vi "CheckSpeedSettings.vi"(2 "TB IP ADDRESS":string="192.168.0.100", 3 "CC IP ADDRESS":string="192.168.0.34", 4 "connection ID CC":refnum<k5>) -> (0 "PASS":bool, 1 "String 2":string)   [LabVIEW 2013]
panel:
  # "INPUTS"
  # "OUTPUTS"
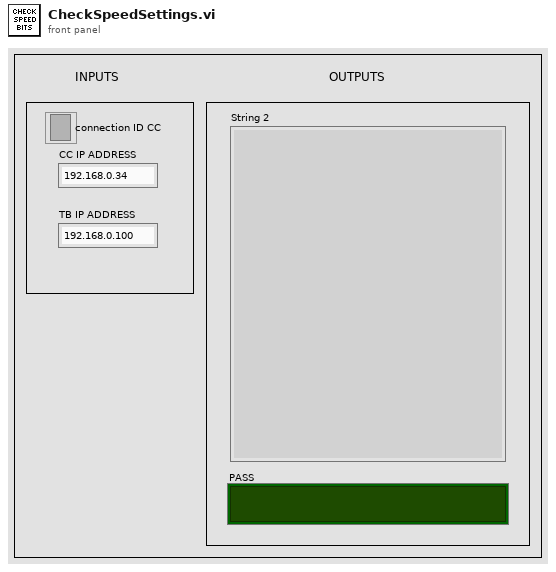
[diagram p1: front panel]
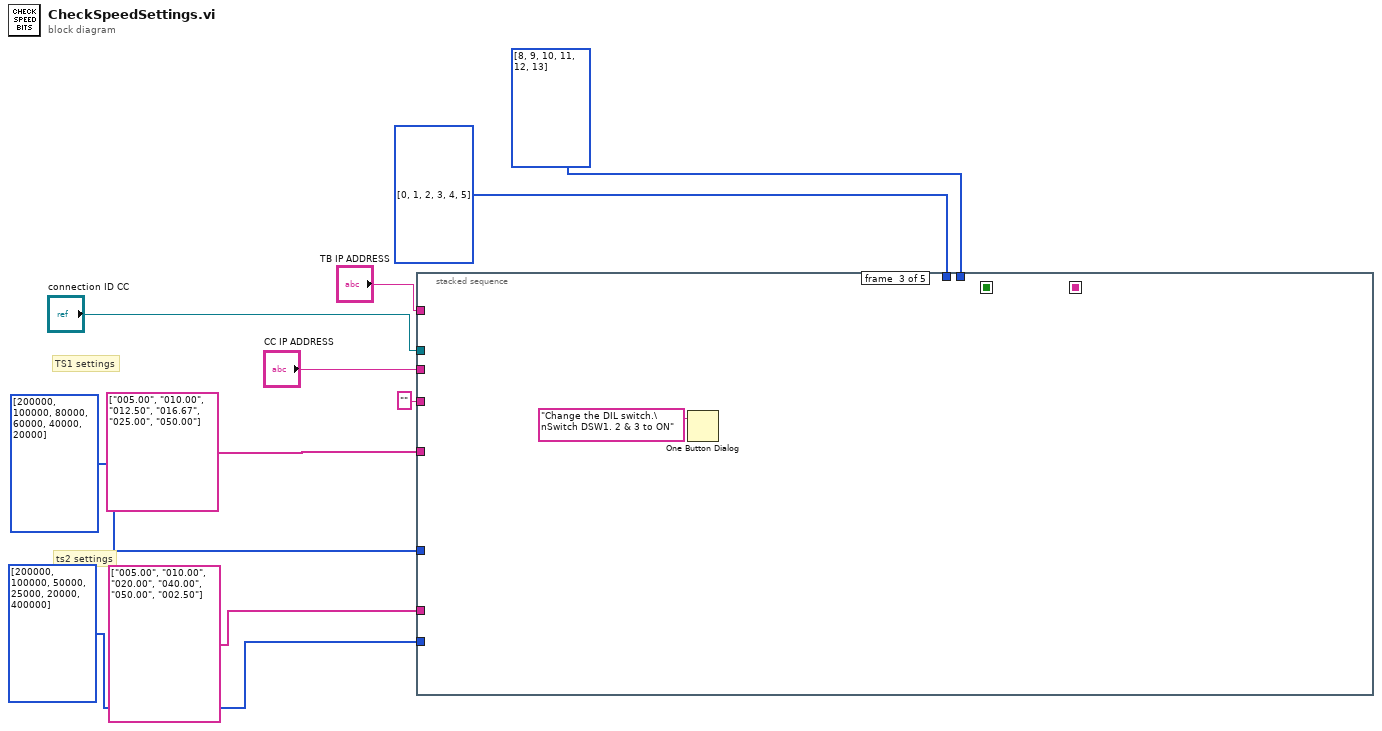
[diagram p0: block diagram]
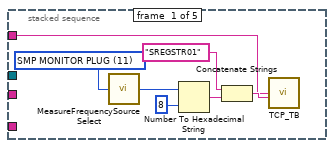
[diagram p2: hidden frame]
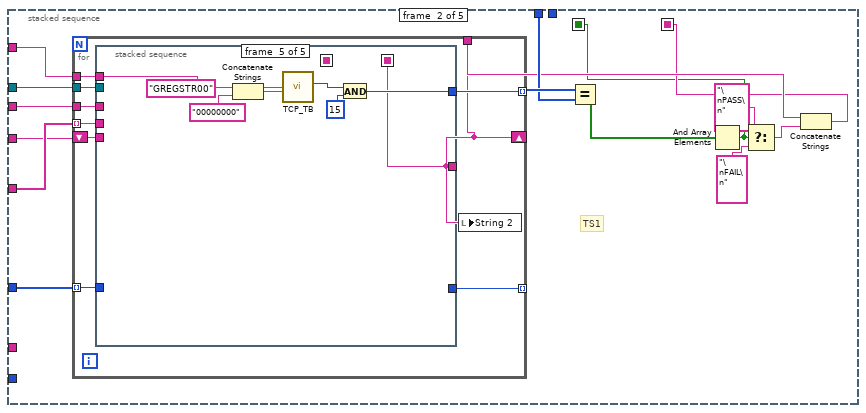
[diagram p3: hidden frame]
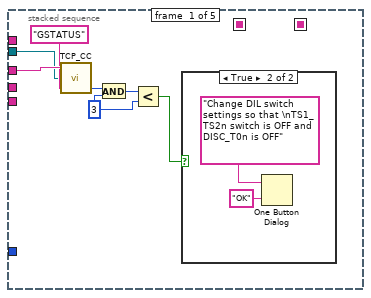
[diagram p4: hidden frame]
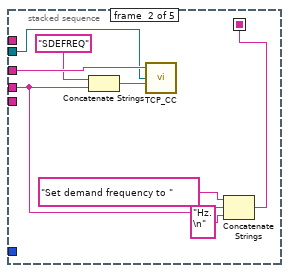
[diagram p6: hidden frame]
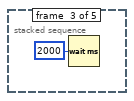
[diagram p7: hidden frame]
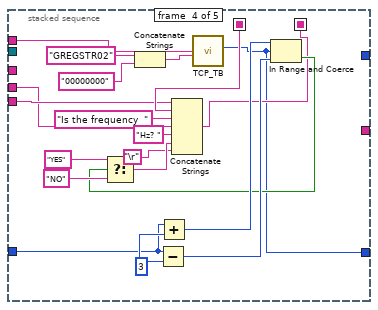
[diagram p8: hidden frame]
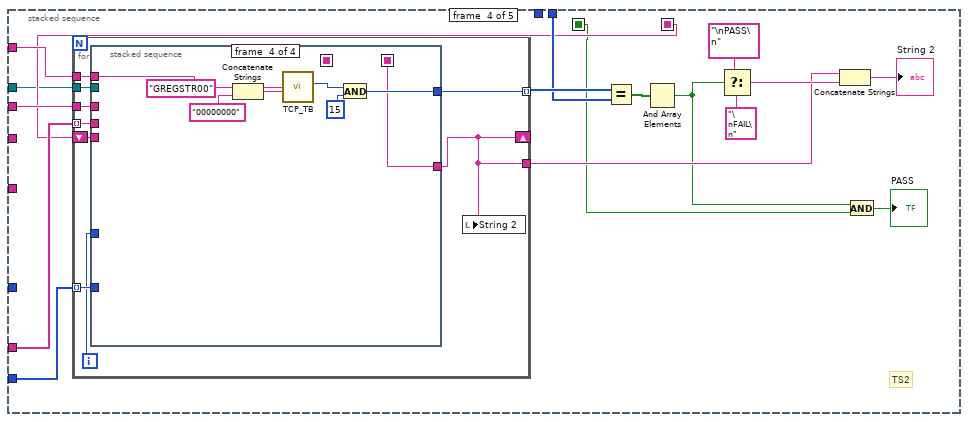
[diagram p9: hidden frame]
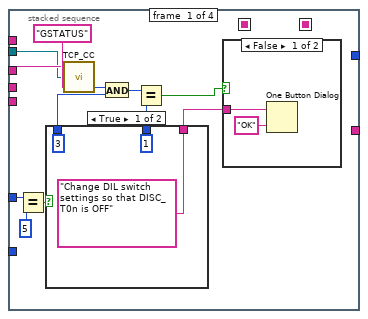
[diagram p10: hidden frame]
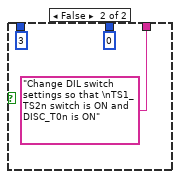
[diagram p11: hidden frame]
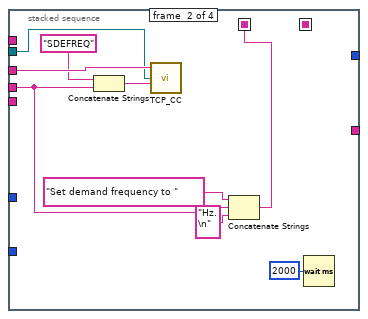
[diagram p13: hidden frame]
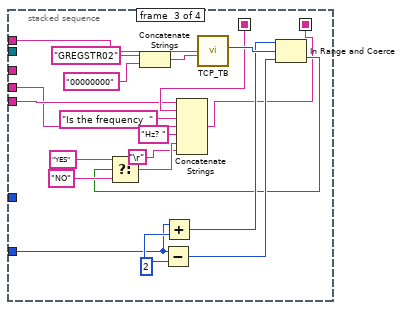
[diagram p14: hidden frame]
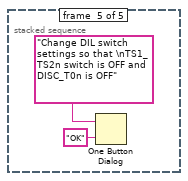
[diagram p15: hidden frame]
diagram:
  # "ts2 settings"
  # "TS1 settings"
  n1 = stacked-sequence {
    seq-local: [_ w20 _ _ _] -> [_ _ _ w99 _]
    seq-local: [_ w19 _ _ _] -> [_ _ _ w91 _]
    tunnel: "CC IP ADDRESS" -> [_ w32 _ w105 _]
    tunnel: "TB IP ADDRESS" -> [w11 w30 _ w104 _]
    tunnel: string[] ["005.00", "010.00", "012.50", "016.67", "025.00", "050.00"] -> [_ w31 _ _ _]
    tunnel: "" ("TB IP ADDRESS") -> [_ w29 _ _ _]
    tunnel: i32[] [200000, 100000, 80000, 60000, 40000, 20000] -> [_ w28 _ _ _]
    tunnel: u32[] [0, 1, 2, 3, 4, 5] ("Array") -> [_ w26 _ _ _]
    tunnel: string[] ["005.00", "010.00", "020.00", "040.00", "050.00", "002.50"] -> [_ _ _ w102 _]
    tunnel: i32[] [200000, 100000, 50000, 25000, 20000, 400000] -> [_ _ _ w101 _]
    tunnel: u32[] [8, 9, 10, 11, 12, 13] ("Array") -> [_ _ _ w100 _]
    tunnel: "connection ID CC" -> [_ w18 _ w89 _]
    frame #0 {
      w13 = u16 11 items=["1Mhz", "1MHz MONITOR PLUG", "DSMP", "DSMP MONITOR PLUG", "RP", "RP MONITOR PLUG", "MP", "MP MONITOR PLUG", "EEP 1.2 Sec", "EEP MONITOR PLUG", "SMP DIFF", "SMP MONITOR PLUG", "SMP Open Collector"] ("Signal Type Select")
      n2 = call "MeasureFrequencySourceSelect.vi"("Signal Type Select"=w13) -> ("Numeric"=w15:i32)
      n3 = Number To Hexadecimal String(1:i16 8 ("width (-)"), 2:w15) -> (0:w16:string)
      n4 = Concatenate Strings("SREGSTR01" ("COMMAND"), w16) -> (w12:string)
      n5 = call "TCP_TB.vi"("IP ADDRESS"=w11, "COMMAND"=w12) -> ()  [unwired: 4 in, 3 out]
    }
    frame #1 {
      # "TS1"
      n6 = for {
        tunnel: w32 -> [w41]
        tunnel: w31 -> [w40] mode=indexing
        tunnel: w30 -> [w39]
        shift-right: [w35] -> _
        shift-left: w29 -> [w38]
        tunnel: w28 -> [w37] mode=indexing
        tunnel: [w36] -> w27 mode=indexing
        tunnel: [w35] -> w21
        tunnel: [w34] -> _ mode=indexing
        tunnel: w18 -> [w33]
        n7 = stacked-sequence {
          seq-local: [_ w52 _ _ _] -> [_ _ _ w66 _]
          seq-local: [_ _ _ w61 _] -> [_ _ _ _ w80]
          tunnel: w41 -> [w48 w58 _ _ _]
          tunnel: w40 -> [_ w54 _ w64 _]
          tunnel: w39 -> [_ _ _ w76 w85]
          tunnel: w38 -> [_ _ _ w65 _]
          tunnel: w37 -> [_ _ _ w62 _]
          tunnel: [_ _ _ _ w81] -> w36
          tunnel: [_ _ _ _ w80] -> w35
          tunnel: [_ _ _ w60 _] -> w34
          tunnel: w33 -> [w42 w51 _ _ _]
          frame #0 {
            w43 = u32 3 ("y")
            n8 = call "TCP_CC.vi"("COMMAND"="GSTATUS", "connection ID"=w42, "IP ADDRESS"=w48) -> ("number"=w46:u32)  [unwired: 2 out]
            n9 = And(x=w46, y=w43) -> (x .and. y?=w45:u32)
            n10 = Less?(x=w45, y=w43) -> (x < y?=w44:bool)
            n11 = case shown="True" w44 {
              frame False {
              }
              frame True {
                n12 = One Button Dialog(message="Change DIL switch settings so that \nTS1_TS2n switch is OFF and DISC_T0n is OFF", button name ("OK")="OK") -> ()  [unwired: 1 out]
              }
            }
          }
          frame #1 {
            n13 = Concatenate Strings("SDEFREQ", w54) -> (w57:string)
            n14 = call "TCP_CC.vi"("COMMAND"=w57, "connection ID"=w51, "IP ADDRESS"=w58) -> ()  [unwired: 3 out]
            n15 = Concatenate Strings("Set demand frequency to ", w54, "Hz.\n" ("string")) -> (w52:string)
          }
          frame #2 {
            n16 = Wait (ms)(milliseconds to wait=u32 2000) -> ()  [unwired: 1 out]
          }
          frame #3 {
            w74 = 3 ("y")
            n17 = Concatenate Strings("GREGSTR02" ("COMMAND"), "00000000" ("string")) -> (w78:string)
            n18 = Subtract(x=w62, y=w74) -> (x-y=w72:i32)
            n19 = Add(x=w62, y=w74) -> (x+y=w73:i32)
            n20 = call "TCP_TB.vi"("IP ADDRESS"=w76, "COMMAND"=w78) -> ("Decinal Number"=w60:u32)  [unwired: 4 in, 2 out]
            n21 = In Range and Coerce(upper limit=w73, x=w60, lower limit=w72) -> (In Range?=w67:bool)  [unwired: 1 out]
            n22 = Select(t="YES" ("string"), s=w67, f="NO" ("string")) -> (s? t:f=w70:string)
            n23 = Concatenate Strings(w65, w66, "Is the frequency  ", w64, "Hz? " ("string"), w70, "\r") -> (w61:string)
          }
          frame #4 {
            n24 = Concatenate Strings("GREGSTR00" ("COMMAND"), "00000000" ("string")) -> (w87:string)
            n25 = call "TCP_TB.vi"("IP ADDRESS"=w85, "COMMAND"=w87) -> ("Decinal Number"=w83:u32)  [unwired: 4 in, 2 out]
            n26 = And(x=w83, y=u32 15) -> (x .and. y?=w81:u32)
          }
        }
        n27 = local write "String 2"(w35) -> ()
      }
      n28 = Equal?(x=w27, y=w26) -> (x = y?=w25:bool[])
      n29 = And Array Elements(Boolean array=w25) -> (logical AND=w19:bool)
      n30 = Select(t="\nPASS\n", s=w19, f="\nFAIL\n") -> (s? t:f=w22:string)
      n31 = Concatenate Strings(w21, w22) -> (w20:string)
    }
    frame #2 {
      n32 = One Button Dialog(message="Change the DIL switch.\nSwitch DSW1. 2 & 3 to ON") -> ()  [unwired: 1 in, 1 out]
    }
    frame #3 {
      # "TS2"
      n33 = for {
        tunnel: w105 -> [w114]
        tunnel: w102 -> [w113] mode=indexing
        tunnel: w104 -> [w112]
        shift-right: [w108] -> _
        shift-left: w99 -> [w111]
        tunnel: w101 -> [w110] mode=indexing
        tunnel: [w109] -> w103 mode=indexing
        tunnel: [w108] -> w93
        tunnel: w89 -> [w106]
        i -> [w107]
        n34 = stacked-sequence {
          seq-local: [_ w136 _ _] -> [_ _ w149 _]
          seq-local: [_ _ w144 _] -> [_ _ _ w164]
          tunnel: w114 -> [w121 w143 _ _]
          tunnel: w113 -> [_ w138 w147 _]
          tunnel: w112 -> [_ _ w160 w169]
          tunnel: w111 -> [_ _ w148 _]
          tunnel: w110 -> [_ _ w145 _]
          tunnel: [_ _ _ w165] -> w109
          tunnel: [_ _ _ w164] -> w108
          tunnel: w107 -> [w119 _ _ _]
          tunnel: w106 -> [w115 w135 _ _]
          frame #0 {
            n35 = Equal?(x=w119, y=5) -> (x = y?=w116:bool)
            n36 = case shown="True" w116 {
              tunnel: [u32 3 ("y") u32 3 ("y")] -> w122
              tunnel: [u32 1 ("y") u32 0 ("y")] -> w120
              tunnel: ["Change DIL switch settings so that DISC_T0n is OFF" ("message") "Change DIL switch settings so that \nTS1_TS2n switch is ON and DISC_T0n is ON" ("message")] -> w117
              frame True {
              }
              frame False {
              }
            }
            n37 = call "TCP_CC.vi"("COMMAND"="GSTATUS", "connection ID"=w115, "IP ADDRESS"=w121) -> ("number"=w125:u32)  [unwired: 2 out]
            n38 = And(x=w125, y=w122) -> (x .and. y?=w124:u32)
            n39 = Equal?(x=w124, y=w120) -> (x = y?=w123:bool)
            n40 = case shown="False" w123 {
              tunnel: w117 -> [w133 _]
              frame False {
                n41 = One Button Dialog(message=w133, button name ("OK")="OK") -> ()  [unwired: 1 out]
              }
              frame True {
              }
            }
          }
          frame #1 {
            n42 = Concatenate Strings("SDEFREQ", w138) -> (w141:string)
            n43 = call "TCP_CC.vi"("COMMAND"=w141, "connection ID"=w135, "IP ADDRESS"=w143) -> ()  [unwired: 3 out]
            n44 = Concatenate Strings("Set demand frequency to ", w138, "Hz.\n" ("string")) -> (w136:string)
            n45 = Wait (ms)(milliseconds to wait=u32 2000) -> ()  [unwired: 1 out]
          }
          frame #2 {
            w157 = 2 ("y")
            n46 = Concatenate Strings("GREGSTR02" ("COMMAND"), "00000000" ("string")) -> (w162:string)
            n47 = Subtract(x=w145, y=w157) -> (x-y=w155:i32)
            n48 = Add(x=w145, y=w157) -> (x+y=w156:i32)
            n49 = call "TCP_TB.vi"("IP ADDRESS"=w160, "COMMAND"=w162) -> ("Decinal Number"=w158:u32)  [unwired: 4 in, 2 out]
            n50 = In Range and Coerce(upper limit=w156, x=w158, lower limit=w155) -> (In Range?=w150:bool)  [unwired: 1 out]
            n51 = Select(t="YES" ("string"), s=w150, f="NO" ("string")) -> (s? t:f=w153:string)
            n52 = Concatenate Strings(w148, w149, "Is the frequency  ", w147, "Hz? " ("string"), w153, "\r") -> (w144:string)
          }
          frame #3 {
            n53 = Concatenate Strings("GREGSTR00" ("COMMAND"), "00000000" ("string")) -> (w171:string)
            n54 = call "TCP_TB.vi"("IP ADDRESS"=w169, "COMMAND"=w171) -> ("Decinal Number"=w167:u32)  [unwired: 4 in, 2 out]
            n55 = And(x=w167, y=u32 15) -> (x .and. y?=w165:u32)
          }
        }
        n56 = local write "String 2"(w108) -> ()
      }
      n57 = Equal?(x=w103, y=w100) -> (x = y?=w95:bool[])
      n58 = And Array Elements(Boolean array=w95) -> (logical AND=w92:bool)
      n59 = Select(t="\nPASS\n", s=w92, f="\nFAIL\n") -> (s? t:f=w96:string)
      n60 = Concatenate Strings(w93, w96) -> (→"String 2":string)
      n61 = And(x=w92, y=w91) -> (x .and. y?=→"PASS":bool)
    }
    frame #4 {
      n62 = One Button Dialog(message="Change DIL switch settings so that \nTS1_TS2n switch is OFF and DISC_T0n is OFF", button name ("OK")="OK") -> ()  [unwired: 1 out]
    }
  }
